vi "led2.vi"() -> ()   [LabVIEW 2014]
panel:
  out "led2":bool
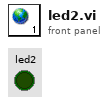
[diagram p1: front panel]
diagram:
